vi "StringParsing.vi"(0 "connection ID":refnum<k5>) -> (2 "State":string, 3 "Flags":string, 4 "P Array":dbl[](array[numeric]), 6 "T Array":dbl[](array[numeric]), 8 "Electrical":dbl[](array[numeric]), 10 "State Variables":dbl[](array[numeric]), 14 "thrust":dbl[](array[numeric]), 15 "valves":dbl[](array[numeric]))   [LabVIEW 2014]
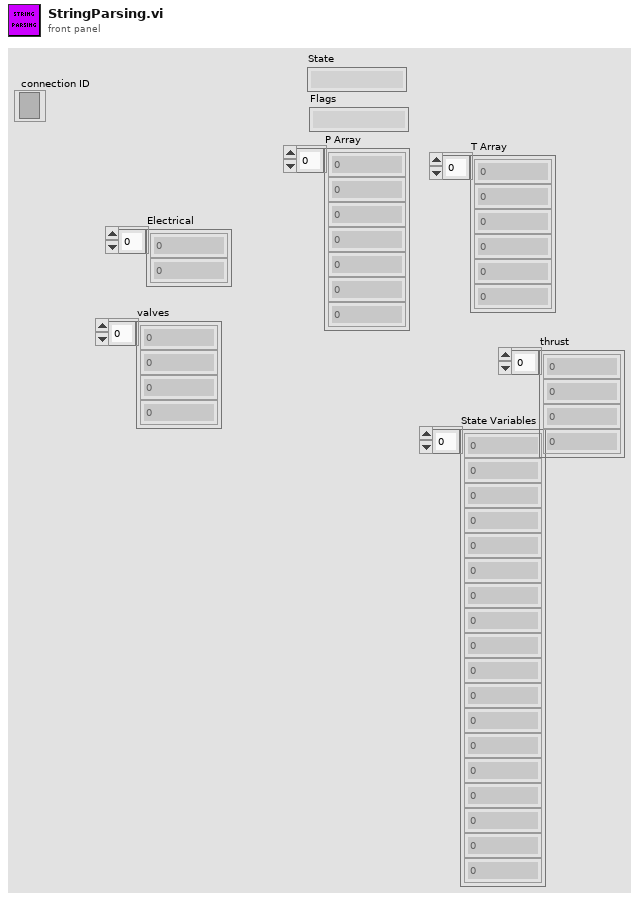
[diagram p1: front panel]
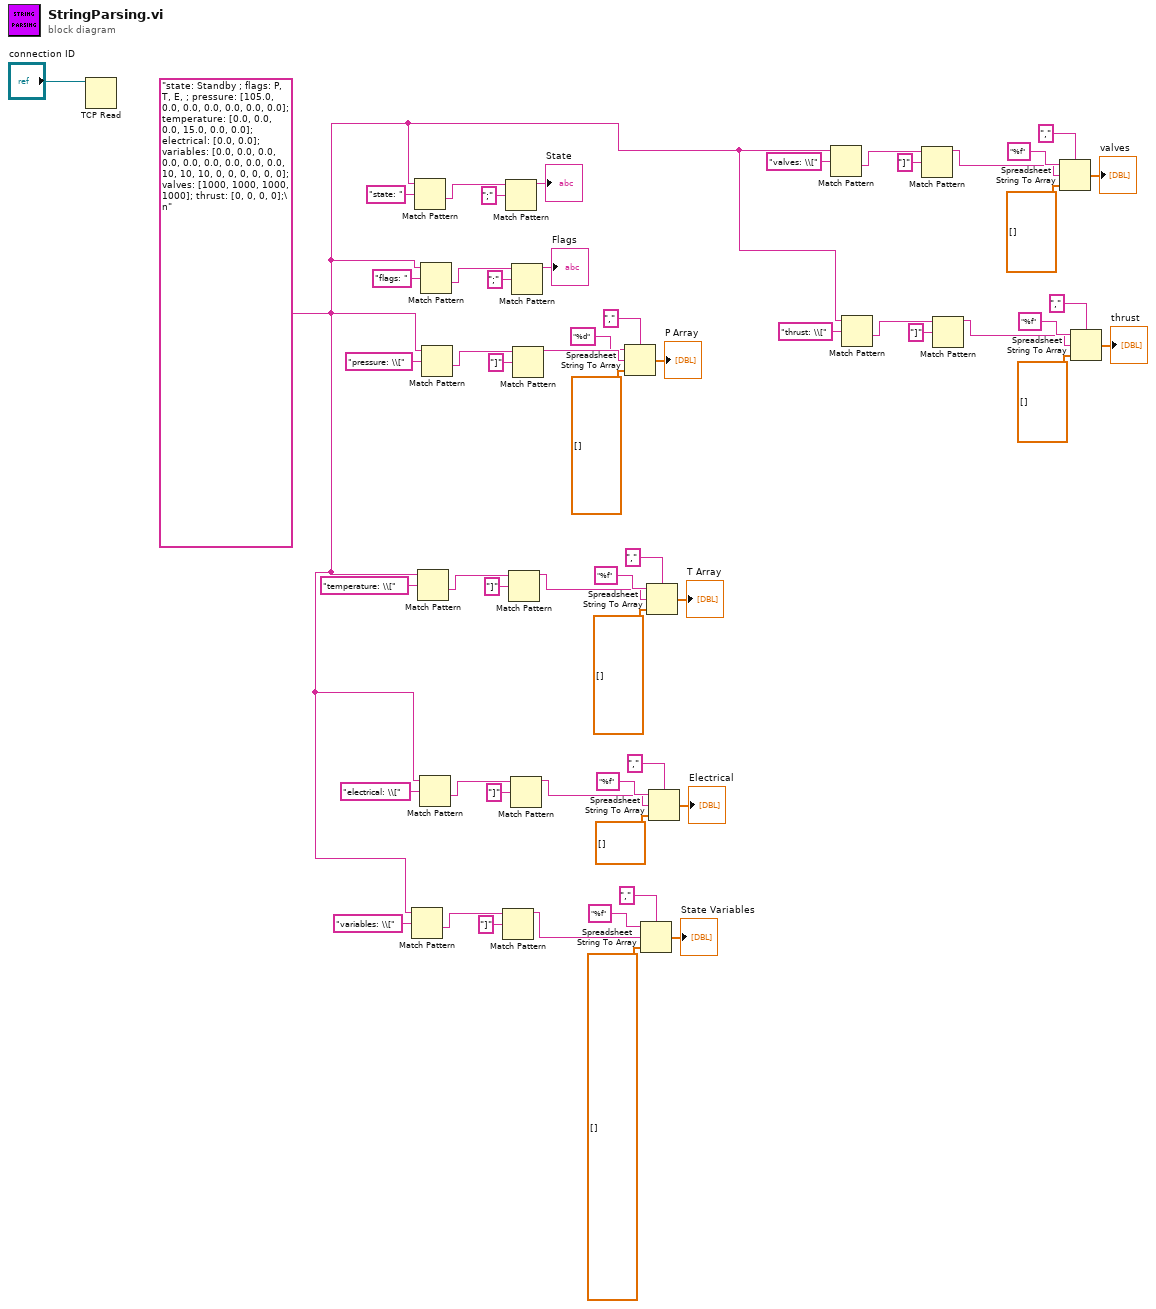
[diagram p0: block diagram]
diagram:
  w1 = "state: Standby ; flags: P, T, E, ; pressure: [105.0, 0.0, 0.0, 0.0, 0.0, 0.0, 0.0]; temperature: [0.0, 0.0, 0.0, 15.0, 0.0, 0.0]; electrical: [0.0, 0.0]; variables: [0.0, 0.0, 0.0, 0.0, 0.0, 0.0, 0.0, 0.0, 0.0, 10, 10, 10, 0, 0, 0, 0, 0, 0]; valves: [1000, 1000, 1000, 1000]; thrust: [0, 0, 0, 0];\n" ("data out")
  n1 = TCP Read(connection ID="connection ID") -> ()  [unwired: 4 in, 3 out]
  n2 = Match Pattern(string=w1, regular expression="variables: \\[") -> (after substring=w24:string)  [unwired: 1 in, 3 out]
  n3 = Match Pattern(string=w1, regular expression="state: ") -> (after substring=w56:string)  [unwired: 1 in, 3 out]
  n4 = Match Pattern(string=w1, regular expression="temperature: \\[") -> (after substring=w40:string)  [unwired: 1 in, 3 out]
  n5 = Match Pattern(string=w1, regular expression="electrical: \\[") -> (after substring=w32:string)  [unwired: 1 in, 3 out]
  n6 = Match Pattern(string=w1, regular expression="flags: ") -> (after substring=w52:string)  [unwired: 1 in, 3 out]
  n7 = Match Pattern(string=w1, regular expression="pressure: \\[") -> (after substring=w42:string)  [unwired: 1 in, 3 out]
  n8 = Match Pattern(string=w24, regular expression="]") -> (before substring=w18:string)  [unwired: 1 in, 3 out]
  n9 = Match Pattern(string=w56, regular expression=";") -> (before substring=→"State":string)  [unwired: 1 in, 3 out]
  n10 = Match Pattern(string=w40, regular expression="]") -> (before substring=w34:string)  [unwired: 1 in, 3 out]
  n11 = Match Pattern(string=w32, regular expression="]") -> (before substring=w26:string)  [unwired: 1 in, 3 out]
  n12 = Match Pattern(string=w52, regular expression=";") -> (before substring=→"Flags":string)  [unwired: 1 in, 3 out]
  n13 = Match Pattern(string=w42, regular expression="]") -> (before substring=w47:string)  [unwired: 1 in, 3 out]
  n14 = Spreadsheet String To Array(delimiter (Tab)=",", format string="%d", spreadsheet string=w47, array type (2D Dbl)=dbl[] []) -> (array=→"P Array":dbl[])
  n15 = Spreadsheet String To Array(delimiter (Tab)=",", format string="%f", spreadsheet string=w18, array type (2D Dbl)=dbl[] []) -> (array=→"State Variables":dbl[])
  n16 = Spreadsheet String To Array(delimiter (Tab)=",", format string="%f", spreadsheet string=w34, array type (2D Dbl)=dbl[] []) -> (array=→"T Array":dbl[])
  n17 = Spreadsheet String To Array(delimiter (Tab)=",", format string="%f", spreadsheet string=w26, array type (2D Dbl)=dbl[] []) -> (array=→"Electrical":dbl[])
  n18 = Match Pattern(string=w1, regular expression="valves: \\[") -> (after substring=w16:string)  [unwired: 1 in, 3 out]
  n19 = Match Pattern(string=w1, regular expression="thrust: \\[") -> (after substring=w8:string)  [unwired: 1 in, 3 out]
  n20 = Match Pattern(string=w16, regular expression="]") -> (before substring=w10:string)  [unwired: 1 in, 3 out]
  n21 = Match Pattern(string=w8, regular expression="]") -> (before substring=w2:string)  [unwired: 1 in, 3 out]
  n22 = Spreadsheet String To Array(delimiter (Tab)=",", format string="%f", spreadsheet string=w10, array type (2D Dbl)=dbl[] []) -> (array=→"valves":dbl[])
  n23 = Spreadsheet String To Array(delimiter (Tab)=",", format string="%f", spreadsheet string=w2, array type (2D Dbl)=dbl[] []) -> (array=→"thrust":dbl[])
